vi "XNET Database Deploy.vi"(0 "IP address":string, 5 "alias":string, 9 "wait for complete? (true)":bool=TRUE, 11 "error in (no error)":errorcluster) -> (10 "percent complete":u32, 15 "error out":errorcluster)   [LabVIEW 2018]
doc: "Deploys a database to a remote LabVIEW Real-Time (RT) target.\n\nIf you need to specify a username and password for the target, use the following syntax for the IP address field:\n\n[<username>:<password>]@<ipaddress>"
uses:
  nixlvapi.dll
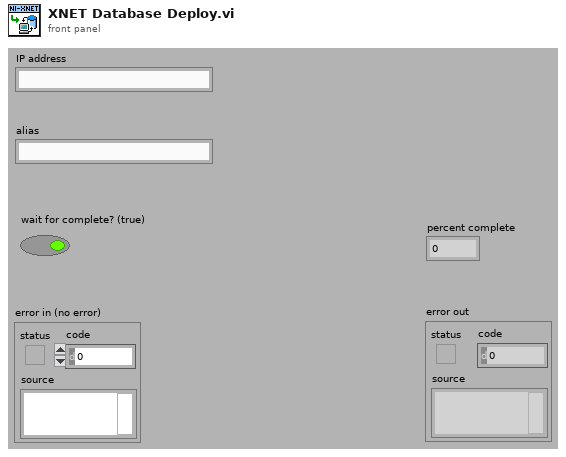
[diagram p1: front panel]
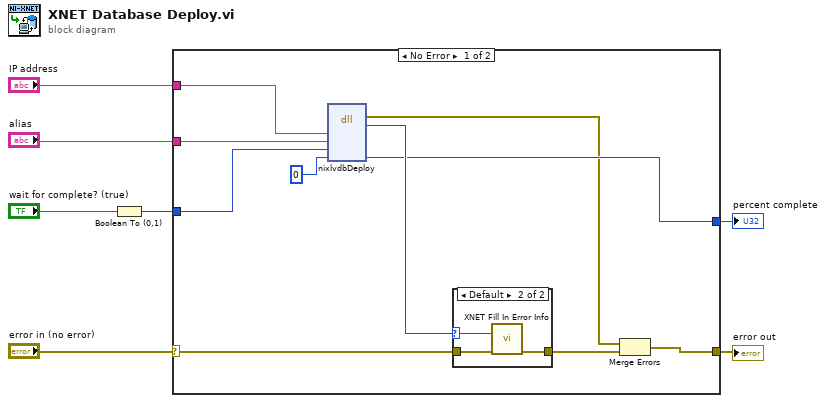
[diagram p0: block diagram]
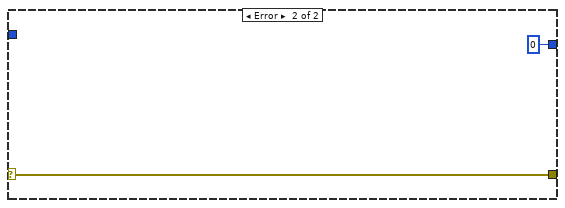
[diagram p3: hidden frame]
diagram:
  n1 = Boolean To (0,1)(Boolean="wait for complete? (true)") -> (0, 1=w2:i16)
  n2 = case shown="No Error" "error in (no error)" {
    selector: "error in (no error)" -> [w16 w23]
    tunnel: "alias" -> [w14 _]
    tunnel: [w9 w23] -> w7
    tunnel: "IP address" -> [w13 _]
    tunnel: w2 -> [w11 _]
    tunnel: [w10 u32 0 ("PercentComplete")] -> w1
    frame No Error {
      n3 = dll-call lib="nixlvapi.*" fn="nixlvdbDeploy" ("nilvxaiu.dll:lvxenDatabaseDeleteObject")("IPAddress"=w13, "DatabaseAlias"=w14, "WaitForComplete"=w11, "PercentComplete"=u32 0) -> (error out=w8:errorcluster, "return type"=w15:i32, "PercentComplete"=w10:u32)  [unwired: 5 in, 2 out]
      n4 = case shown="Default" w15 {
        selector: w15 -> [_ w19]
        tunnel: w16 -> [w18 w20]
        tunnel: [w18 w21] -> w17
        frame 0 {
        }
        frame Default {
          n5 = call "XNET Fill In Error Info.vi"("status code"=w19, "error in"=w20) -> ("error out"=w21:errorcluster)  [unwired: 13 out]
        }
      }
      n6 = Merge Errors(w8, w17) -> (w9:errorcluster)
    }
    frame Error {
    }
  }
  "error out" <- w7
  "percent complete" <- w1
